vi "Get SLSC Switch Reservation Group.vi"(8 "error in":errorcluster, 11 "slsc switch custom device in":T1 format="%.0x") -> (0 "error out":errorcluster, 1 "default value?":bool, 2 "reservation group":string, 3 "slsc switch custom device out":T1 format="%.0x")   [LabVIEW 2017, in "NI-SWITCH Scripting.lvlib"]
doc: "Returns the configured reservation group for the SLSC Switch custom device."
uses:
  NI-SWITCH Scripting.lvlib
  <vilib>/NI Veristand/Custom Device API/Custom Device Item Ref.ctl
  SLSC Scripting Constants.vi
  <vilib>/NI Veristand/Custom Device API/Get Item Property (String).vi
  <vilib>/NI VeriStand/Custom Device API/Custom Device API.lvlib
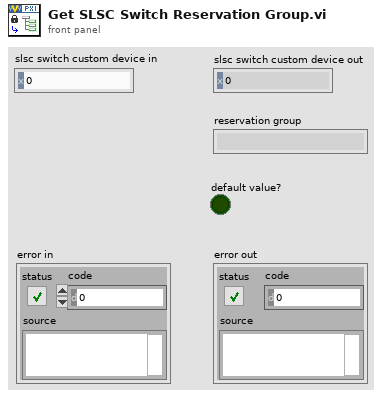
[diagram p1: front panel]
types:
  T1 = typedef "Custom Device API.lvlib/Custom Device Item Ref.ctl" = u64
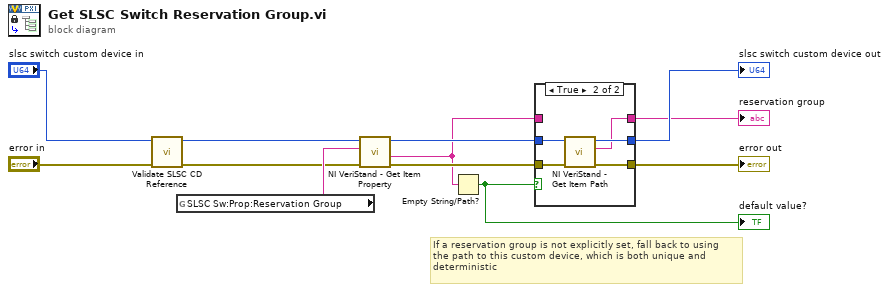
[diagram p0: block diagram]
diagram:
  # "If a reservation group is not explicitly set, fall back to using\nthe path to this custom device, which is both unique and\ndeterministic"
  n1 = call "Validate SLSC CD Reference.vi"("error in"="error in", "slsc switch custom device in"="slsc switch custom device in") -> ("error out"=w10:errorcluster, "slsc switch custom device out"=w8:T1)  [unwired: 8 in]
  n2 = global read "SLSC Scripting Constants.vi" "SLSC Sw:Prop:Reservation Group"() -> (w12:string)
  n3 = call-poly <vilib>:"NI VeriStand - Get Item Property.vi"("error in (no error)"=w10, "Property Name"=w12, "Item Ref in"=w8) -> ("error out"=w6:errorcluster, "Value"=w1:string, "Item Ref out"=w4:T1)  [unwired: 5 in, 1 out]
  n4 = Empty String/Path?(string/path=w1) -> (empty?=w5:bool)
  "default value?" <- w5
  n5 = case shown="True" w5 {
    tunnel: [w14 w19] -> w3
    tunnel: w4 -> [w14 w20]
    tunnel: w6 -> [w15 w17]
    tunnel: [w15 w18] -> w7
    tunnel: [w13 w16] -> w2
    tunnel: w1 -> [w13 _]
    frame False {
    }
    frame True {
      n6 = call <vilib>:"NI VeriStand - Get Item Path.vi"("error in (no error)"=w17, "Item Ref in"=w20) -> ("error out"=w18:errorcluster, "Path"=w16:string, "Item Ref out"=w19:T1)  [unwired: 6 in, 1 out]
    }
  }
  "error out" <- w7
  "slsc switch custom device out" <- w3
  "reservation group" <- w2
